vi "RH_DCPower_0V_Stop.vi"(8 "error in (no error)":errorcluster, 9 "milliseconds to wait":dbl=100.0, 10 "Channel List":string, 11 "DCPower Session In":refnum<k15>) -> (0 "error out":errorcluster, 3 "DCPower Session Out":refnum<k15>)   [LabVIEW 2023, in "ResourceHandling.lvlib"]
doc: "Set the voltage level to 0V, waits a certain amount of time before stopping and disabling the output"
uses:
  ResourceHandling.lvlib
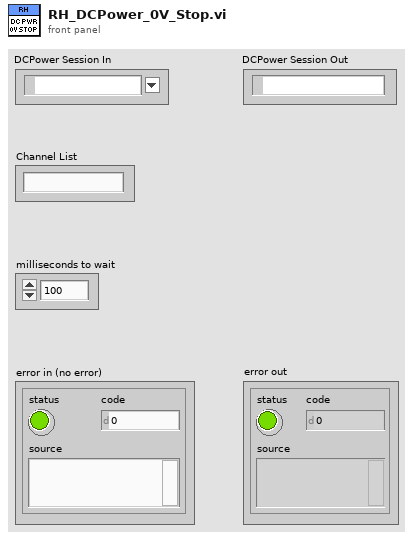
[diagram p1: front panel]
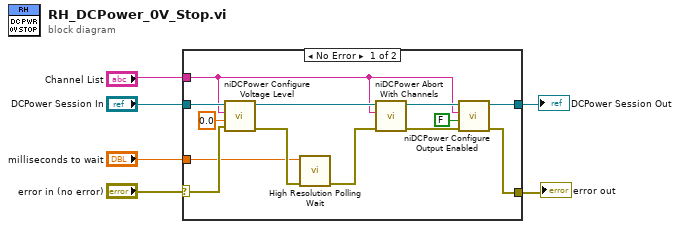
[diagram p0: block diagram]
diagram:
  n1 = case shown="No Error" "error in (no error)" {
    selector: "error in (no error)" -> [w12 w20]
    tunnel: [w19 w21] -> w2
    tunnel: "DCPower Session In" -> [w18 w21]
    tunnel: "Channel List" -> [w11 _]
    tunnel: "milliseconds to wait" -> [w7 _]
    tunnel: [w10 w20] -> w1
    frame No Error {
      n2 = call <instrlib>:"niDCPower Configure Voltage Level.vi"("error in (no error)"=w12, "voltage level"=0.0, "channel name"=w11, "instrument handle"=w18) -> ("error out"=w9:errorcluster, "instrument handle out"=w13:refnum<k15>)  [unwired: 6 in]
      n3 = call <vilib>:"High Resolution Polling Wait.vi"("error in (no error)"=w9, "seconds to wait"=w7) -> ("error out"=w8:errorcluster)  [unwired: 9 in]
      n4 = call <instrlib>:"niDCPower Abort With Channels.vi"("error in (no error)"=w8, "channel name"=w11, "instrument handle"=w13) -> ("error out"=w17:errorcluster, "instrument handle out"=w16:refnum<k15>)  [unwired: 7 in]
      n5 = call <instrlib>:"niDCPower Configure Output Enabled.vi"("error in (no error)"=w17, "output enabled"=FALSE, "channel name"=w11, "instrument handle"=w16) -> ("error out"=w10:errorcluster, "instrument handle out"=w19:refnum<k15>)  [unwired: 6 in]
    }
    frame Error {
    }
  }
  "DCPower Session Out" <- w2
  "error out" <- w1
